vi "modify channel test.vi"() -> ()   [LabVIEW 2013, in "Shared Library Module tests.lvlib"]
doc: "Platypus Framework 1.0.1.60\nNI Systems Engineering - National Instruments"
uses:
  Shared Library Module tests.lvlib
  <vilib>/NI/Tag Bus Module Framework/channel/channel classification.ctl
  configuration/Shared Library Module configuration.lvclass
  <vilib>/NI/Tag Bus Module Framework/channel/TBM channel.lvclass/TBM channel.ctl
  <vilib>/NI/Tag Bus/tag/tag descriptor.lvclass/tag descriptor.ctl
  <vilib>/NI/Tag Bus Module Framework/channel/Read channel classification.vi
  <vilib>/NI/Tag Bus Module Framework/channel/Write channel classification.vi
  <vilib>/NI/Tag Bus/tag/read tag name.vi
  <vilib>/NI/Tag Bus Module Framework/channel/TBM channel.lvclass
  <vilib>/NI/Tag Bus Module Framework/root configuration/TBM configuration.lvclass
panel:
  out "rename success":bool
  out "no err":errorcluster
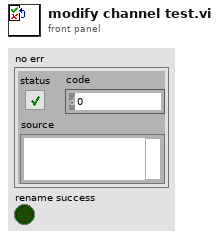
[diagram p1: front panel]
types:
  T1 = typedef "TBM channel.lvclass/channel classification.ctl" = enum16{"input data", "output data", "processing parameter", "processing result"}
  T2 = typedef "tag bus.lvlib/tag descriptor.lvclass/Data Type.ctl" = enum16{"Double", "Single", "I64", "I32", "I16", "I8", "U64", "U32", "U16", "U8", "Boolean", "String", "Array of Double", "Array of Single", "Array of I64", "Array of I32", "Array of I16", "Array of I8", "Array of U64", "Array of U32", "Array of U16", "Array of U8", "Array of Boolean", "Array of String"}
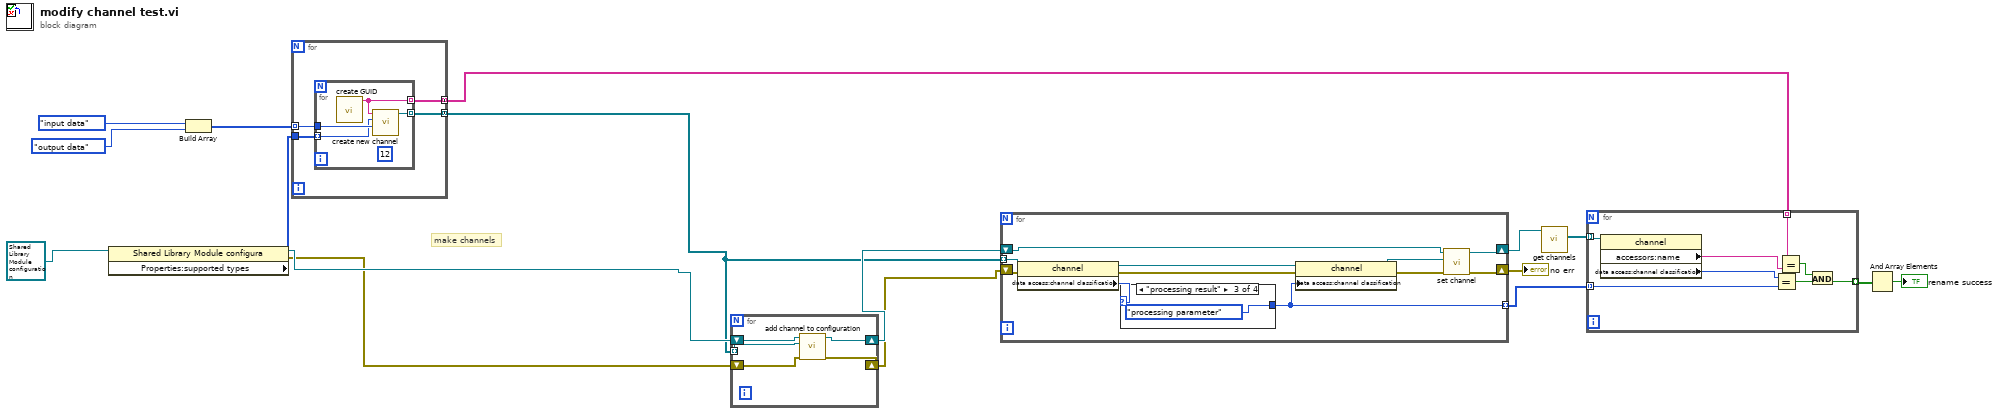
[diagram p0: block diagram]
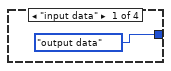
[diagram p2: hidden frame]
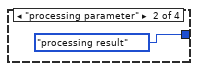
[diagram p3: hidden frame]
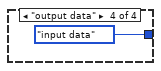
[diagram p4: hidden frame]
diagram:
  # "make channels"
  n1 = property class="Shared Library Module configura"(reference=refnum<class "Shared Library Module configuration.lvclass"> refnum ("tag bus configurable plugin module configuration")) -> (reference out=w5:refnum<class "Shared Library Module configuration.lvclass">, error out=w1:errorcluster, "Properties:supported types"=w14:T2[])  [unwired: 1 in]
  n2 = Build Array(channel_classification."input data" ("channel classification"), channel_classification."output data" ("channel classification")) -> (w15:T1[])
  n3 = for {
    tunnel: w15 -> [w21] mode=indexing
    tunnel: [w19] -> w3 mode=concatenating
    tunnel: w14 -> [w20]
    tunnel: [w18] -> w7 mode=concatenating
    n4 = for {
      tunnel: w21 -> [w24]
      tunnel: [w25] -> w19 mode=indexing
      tunnel: w20 -> [w23] mode=indexing
      tunnel: [w22] -> w18 mode=indexing
      (unwired) 12
      n5 = call <vilib>:"create GUID.vi"() -> ("uuid"=w22:string)  [unwired: 11 in]
      n6 = call <vilib>:"create new channel.vi"("channel classification"=w24, "data type"=w23, "channel name"=w22) -> ("channel"=w25:refnum<class "TBM channel.lvclass">)  [unwired: 8 in]
    }
  }
  n7 = for {
    shift-right: [w29] -> w4
    shift-left: w5 -> [w30]
    shift-right: [w28] -> w2
    shift-left: w1 -> [w27]
    tunnel: w3 -> [w26] mode=indexing
    n8 = call "add channel to configuration.vi"("error in"=w27, "TBM channel in"=w26, "Shared Library Module configuration in"=w30) -> ("error out"=w28:errorcluster, "Shared Library Module configuration out"=w29:refnum<class "Shared Library Module configuration.lvclass">)  [unwired: 7 in]
  }
  n9 = for {
    shift-right: [w40] -> w13
    shift-left: w4 -> [w41]
    shift-right: [w39] -> w12
    shift-left: w2 -> [w38]
    tunnel: w3 -> [w36] mode=indexing
    tunnel: [w31] -> w8 mode=indexing
    n10 = property class="channel"(reference=w36, error in=w38) -> (reference out=w34:refnum<class "TBM channel.lvclass">, error out=w37:errorcluster, "data access:channel classification"=w32:T1)
    n11 = case shown="\"processing result\"" w32 {
      tunnel: [channel_classification."output data" ("channel classification") channel_classification."processing result" ("channel classification") channel_classification."processing parameter" ("channel classification") channel_classification."input data" ("channel classification")] -> w31
      frame "input data" {
      }
      frame "processing parameter" {
      }
      frame "processing result" {
      }
      frame "output data" {
      }
    }
    n12 = property class="channel"(reference=w34, error in=w37, "data access:channel classification"=w31) -> (reference out=w33:refnum<class "TBM channel.lvclass">, error out=w35:errorcluster)
    n13 = call "set channel.vi"("error in"=w35, "TBM channel in"=w33, "Shared Library Module configuration in"=w41) -> ("error out"=w39:errorcluster, "Shared Library Module configuration out"=w40:refnum<class "Shared Library Module configuration.lvclass">)  [unwired: 7 in]
  }
  "no err" <- w12
  n14 = call-dynamic "get channels.vi"("Shared Library Module configuration in"=w13) -> ("channels"=w11:refnum<class "TBM channel.lvclass">[])  [unwired: 9 in, 1 out]
  n15 = for {
    tunnel: w11 -> [w52] mode=indexing
    tunnel: [w51] -> w10 mode=indexing
    tunnel: w8 -> [w50] mode=indexing
    tunnel: w7 -> [w47] mode=indexing
    n16 = property class="channel"(reference=w52) -> ("accessors:name"=w48:string, "data access:channel classification"=w49:T1)  [unwired: 1 in, 2 out]
    n17 = Equal?(x=w49, y=w50) -> (x = y?=w53:bool)
    n18 = Equal?(x=w47, y=w48) -> (x = y?=w46:bool)
    n19 = And(x=w46, y=w53) -> (x .and. y?=w51:bool)
  }
  n20 = And Array Elements(Boolean array=w10) -> (logical AND=→"rename success":bool)
